vi "Arduino Start Comms.vi"(1 "Resource index":i32, 2 "VISA resource name":refnum<visa-resource-name>, 3 "Arduino VISA config & resource":T1={"baud rate (bps)"=276000, "timeout (ms)"=12000, "data bits"=8, "parity"=enum."None", "stop bits (10: 1 bit)"=10, "flow control"=0, "termination char (hex)"=10, "Enable Termination Char"=FALSE, "byte count"=12, "Resource locked?"=FALSE} {"termination char (hex)" format="%02x"; "stop bits (10: 1 bit)" items=["1.0"=10, "1.5"=15, "2.0"=20]; "flow control" items=["None", "XON/XOFF", "RTS/CTS", "XON/XOFF & RTS/CTS", "DTR/DSR", "XON/XOFF & DTR/DSR"]}) -> (0 "Error":errorcluster)   [LabVIEW 2018]
uses:
  ctls_and_globals/Arduino Config & resource typedef.ctl
  <vilib>/Instr/_visa.llb/VISA Open Access Mode.ctl
  ctls_and_globals/Arduino Global.vi
  <vilib>/Instr/_visa.llb/VISA Configure Serial Port (Instr).vi
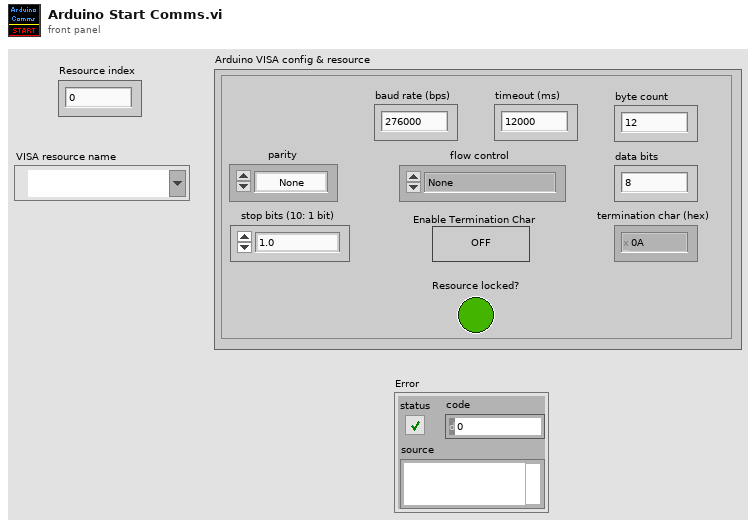
[diagram p1: front panel]
types:
  T1 = typedef "Arduino Config & resource typedef.ctl" = cluster{"baud rate (bps)":u32, "timeout (ms)":u32, "data bits":u16, "parity":enum16{"None", "Odd", "Even", "Mark", "Space"}, "stop bits (10: 1 bit)":u16, "flow control":u16, "termination char (hex)":u8, "Enable Termination Char":bool, "byte count":u32, "Resource locked?":bool}
  T2 = typedef "VISA Open Access Mode.ctl" = u32
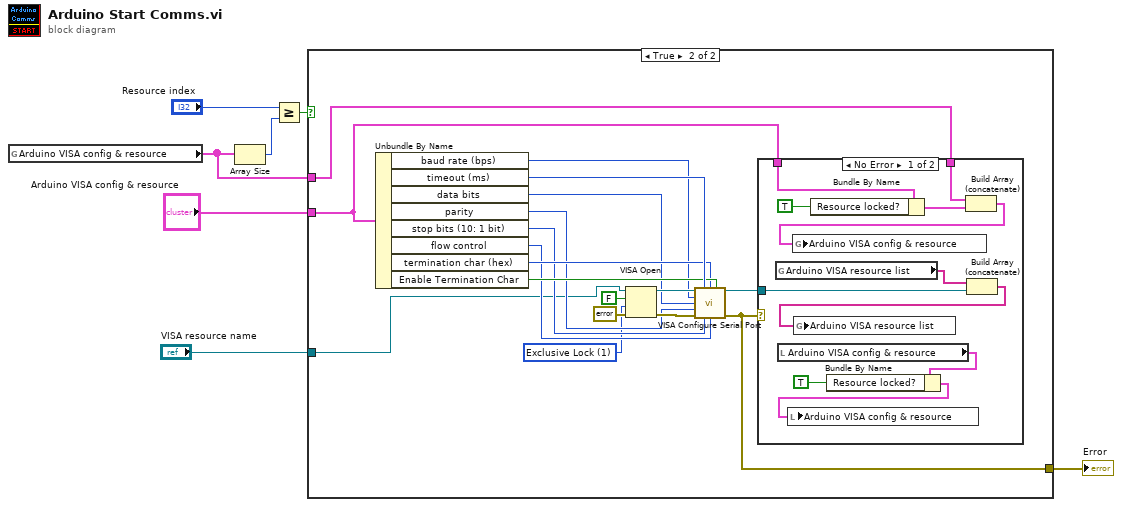
[diagram p0: block diagram]
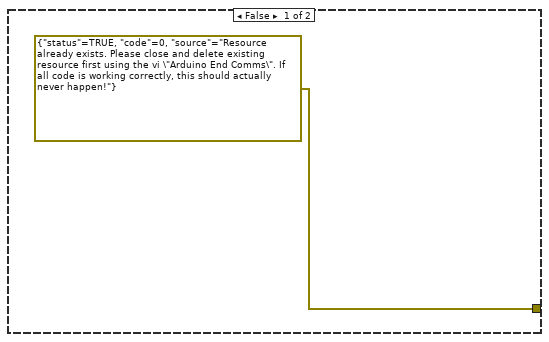
[diagram p2: hidden frame]
diagram:
  n1 = global read "Arduino Global.vi" "Arduino VISA config & resource"() -> (w5:T1[])
  n2 = Array Size(array=w5) -> (size(s)=w7:i32)
  n3 = Greater Or Equal?(x="Resource index", y=w7) -> (x >= y?=w6:bool)
  n4 = case shown="True" w6 {
    tunnel: w5 -> [_ w14]
    tunnel: "Arduino VISA config & resource" -> [_ w15]
    tunnel: [errorcluster {"status"=TRUE, "code"=0, "source"="Resource already exists. Please close and delete existing resource first using the vi \"Arduino End Comms\". If all code is working correctly, this should actually never happen!"} ("error out") w10] -> w3
    tunnel: "VISA resource name" -> [_ w9]
    frame False {
    }
    frame True {
      w12 = T2 1 items=["VISA Defaults"=0, "Exclusive Lock"=1, "Load Configured Settings"=4] ("Access Mode")
      n5 = Unbundle By Name(w15) -> ("baud rate (bps)"=w20:u32, "timeout (ms)"=w23:u32, "data bits"=w19:u16, "parity"=w18:enum16{"None", "Odd", "Even", "Mark", "Space"}, "stop bits (10: 1 bit)"=w17:u16, "flow control"=w16:u16, "termination char (hex)"=w21:u8, "Enable Termination Char"=w22:bool)
      n6 = VISA Open(duplicate session (F)=FALSE, access mode=w12, error in (no error)=errorcluster {"status"=FALSE, "code"=0, "source"=""}, VISA resource name=w9) -> (VISA resource name=w25:refnum<visa-resource-name>, error out=w26:errorcluster)  [unwired: 1 in]
      n7 = call-poly "VISA Configure Serial Port"("VISA resource name"=w25, "timeout (10sec)"=w23, "termination char\n(0xA = '\\n' = LF)"=w21, "Enable Termination\nChar (T)"=w22, "baud rate (9600)"=w20, "data bits (8)"=w19, "parity (0:none)"=w18, "error in (no error)"=w26, "stop bits (10: 1 bit)"=w17, "flow control (0:none)"=w16) -> ("VISA resource name out"=w11:refnum<visa-resource-name>, "error out"=w10:errorcluster)  [unwired: 4 in]
      n8 = case shown="No Error" w10 {
        tunnel: w15 -> [w37 _]
        tunnel: w14 -> [w34 _]
        tunnel: w11 -> [w28 _]
        frame No Error {
          n9 = global read "Arduino Global.vi" "Arduino VISA resource list"() -> (w29:string[])
          n10 = local read "Arduino VISA config & resource"() -> (w31:T1)
          n11 = Bundle By Name(cluster=w37, "Resource locked?"=TRUE) -> (w35:T1)
          n12 = Bundle By Name(cluster=w31, "Resource locked?"=TRUE) -> (w30:T1)
          n13 = local write "Arduino VISA config & resource"(w30) -> ()
          n14 = Build Array (concatenate)(w34, w35) -> (w33:T1[])
          n15 = global write "Arduino Global.vi" "Arduino VISA config & resource"(w33) -> ()
          n16 = Build Array (concatenate)(w29, w28) -> (w27:string[])
          n17 = global write "Arduino Global.vi" "Arduino VISA resource list"(w27) -> ()
        }
        frame Error {
        }
      }
    }
  }
  "Error" <- w3
